vi "Test1_5b.vi"(0 "Instrument VISA in":T1={"AWG VISA"="81160A", "Oscilloscope  VISA "="DSO80204B", "Integration Board IP"="172.16.7.43", "connection ID"=refnum, "report out"=refnum}, 2 "Report Enable":bool, 5 "L1 version":bool, 9 "Cycles Burst":i32=10000, 11 "error in":errorcluster) -> (4 "Instrument VISA out":T1={"AWG VISA"="81160A", "Oscilloscope  VISA "="DSO80204B", "Integration Board IP"="172.16.7.43", "connection ID"=refnum, "report out"=refnum}, 6 "DT_50_L0":i32[][](array[numeric]), 8 "L1 Level Above Noise":i32, 15 "error out":errorcluster)   [LabVIEW 2009]
doc: "This VI helps in the comparison between the sum of different channels."
uses:
  <instrlib>/Agilent 81150/Agilent 81150.lvlib
  <vilib>/Analysis/NI_AALPro.lvlib
  <vilib>/Utility/NIReport.llb/NI_report.lvclass
panel:
  out "XY Graph":cluster{"Y":dbl[], "Y":dbl[]}[](graph)
  out "IPR_Address":i32
  out "L1 Address":i32=17
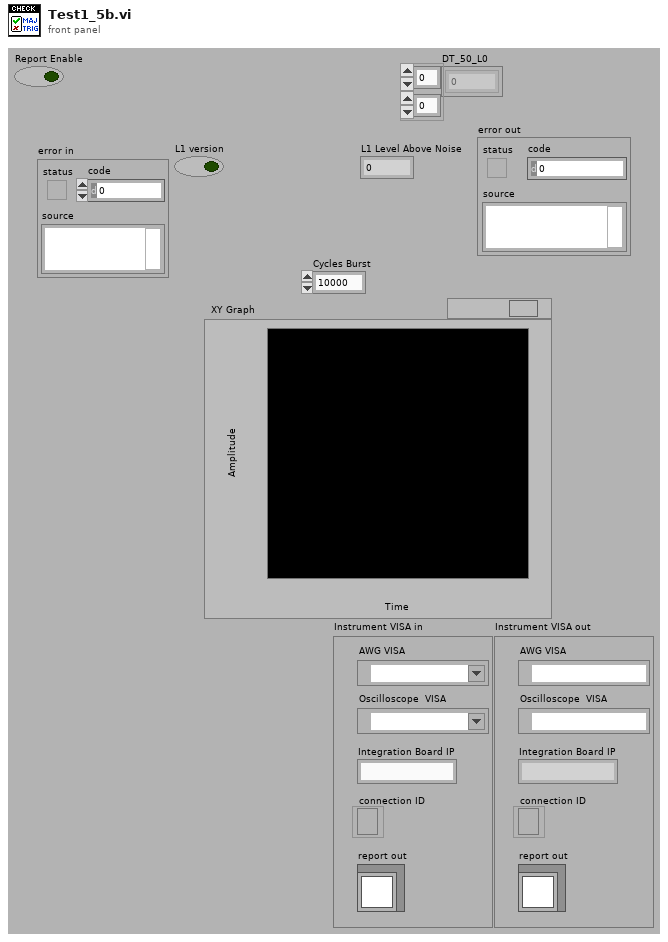
[diagram p1: front panel]
types:
  T1 = cluster{"AWG VISA":refnum<visa-resource-name>, "Oscilloscope  VISA ":refnum<visa-resource-name>, "Integration Board IP":string, "connection ID":refnum<k5>, "report out":refnum<class "NI_report.lvclass">}
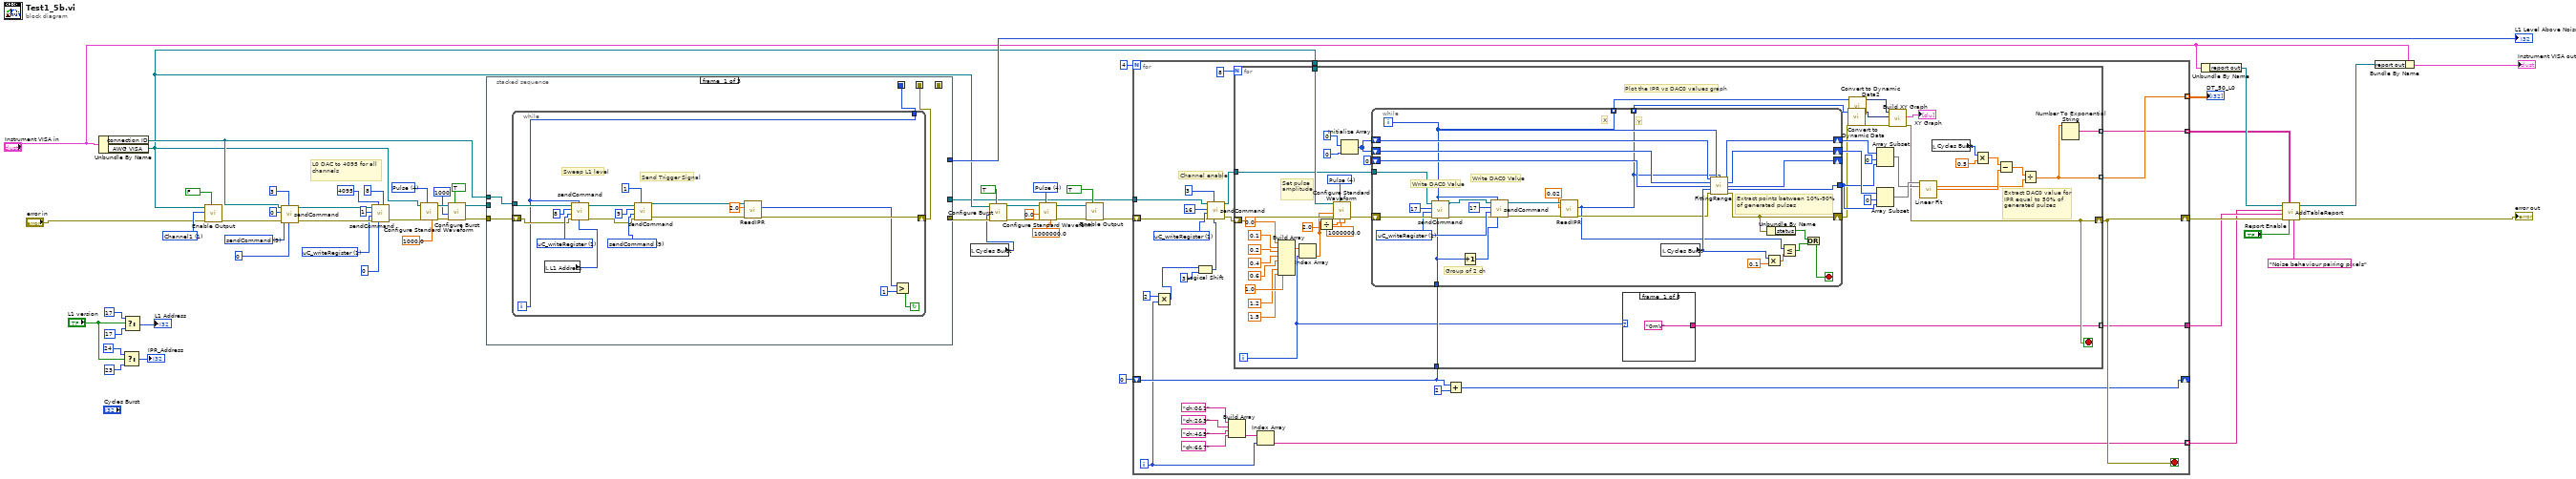
[diagram p0: block diagram]
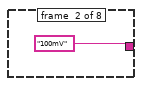
[diagram p2: hidden frame]
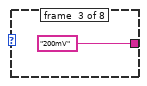
[diagram p3: hidden frame]
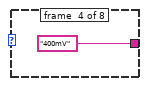
[diagram p4: hidden frame]
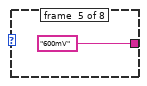
[diagram p5: hidden frame]
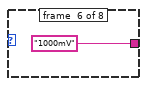
[diagram p6: hidden frame]
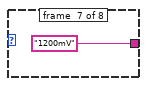
[diagram p7: hidden frame]
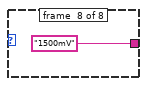
[diagram p8: hidden frame]
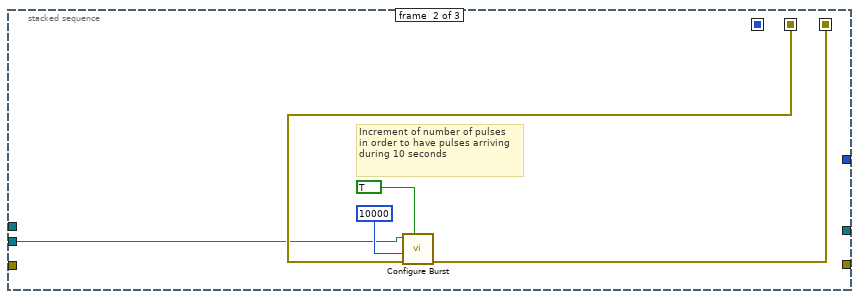
[diagram p9: hidden frame]
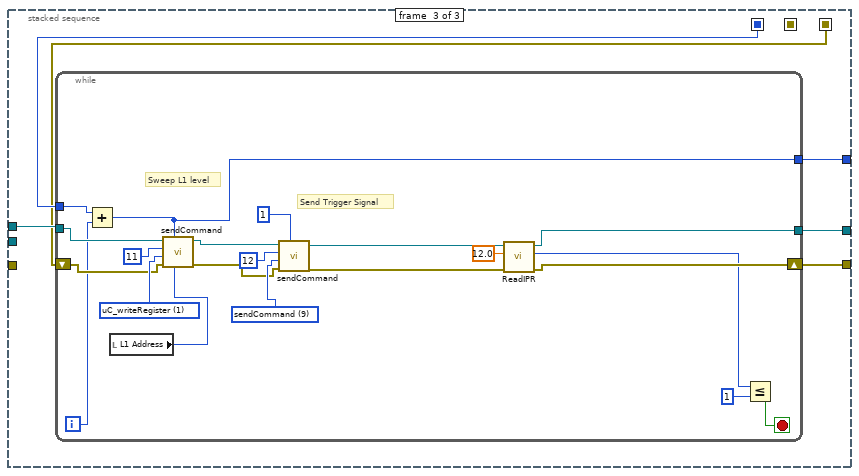
[diagram p10: hidden frame]
diagram:
  w28 = u16 4 items=["Sine", "Square", "Ramp Up", "Ramp Down", "Pulse", "Noise", "DC"] ("Waveform (0: Sine)")
  w44 = u16 4 items=["Sine", "Square", "Ramp Up", "Ramp Down", "Pulse", "Noise", "DC"] ("Waveform (0: Sine)")
  w51 = u16 1 items=["sendCommand"=9, "FPGA_writeRegister"=3, "FPGA_readRegister"=2, "uC_writeRegister"=1, "uC_readRegister"=0] ("Action")
  w58 = u16 9 items=["sendCommand"=9, "FPGA_writeRegister"=3, "FPGA_readRegister"=2, "uC_writeRegister"=1, "uC_readRegister"=0] ("Action")
  w60 = u16 1 items=["Channel1"=1, "Channel2"=2] ("Channel (1: Channel1)")
  # "L0 DAC to 4095 for all channels"
  n1 = Unbundle By Name("Instrument VISA in") -> ("connection ID"=w39:refnum<k5>, "AWG VISA"=w29:refnum<visa-resource-name>)
  n2 = Select(t=24 ("Address"), s="L1 version", f=23 ("Address")) -> (s? t:f=→"IPR_Address":i32)
  n3 = Select(t=17 ("Address"), s="L1 version", f=17 ("Address")) -> (s? t:f=→"L1 Address":i32)
  n4 = call <instrlib>:"Enable Output.vi"("Enable Output (T: Enable)"=FALSE, "error in (no error)"="error in", "Channel (1: Channel1)"=w60, "VISA resource name"=w29) -> ("error out"=w57:errorcluster)  [unwired: 6 in, 1 out]
  n5 = call "sendCommand.vi"("Address"=0, "Data"=3, "error in"=w57, "Action"=w58, "id_in"=0 ("id"), "connection ID"=w39) -> ("error out"=w53:errorcluster, "connection ID out"=w52:refnum<k5>)  [unwired: 1 in, 3 out]
  n6 = call "sendCommand.vi"("number data"=8, "Address"=0, "Data"=4095, "error in"=w53, "Action"=w51, "id_in"=1 ("id"), "connection ID"=w52) -> ("error out"=w46:errorcluster)  [unwired: 4 out]
  n7 = call <instrlib>:"Configure Standard Waveform.vi"("Frequency (1000.0 Hz)"=1000.0, "Waveform (0: Sine)"=w44, "error in (no error)"=w46, "VISA resource name"=w29) -> ("error out"=w43:errorcluster, "VISA resource name out"=w42:refnum<visa-resource-name>)  [unwired: 6 in]
  n8 = call <instrlib>:"Configure Burst.vi"("Enable Burst (F: Disable)"=TRUE, "error in (no error)"=w43, "Burst Count (2)"=1000, "VISA resource name"=w42) -> ("error out"=w40:errorcluster, "VISA resource name out"=w38:refnum<visa-resource-name>)  [unwired: 6 in]
  n9 = stacked-sequence {
    seq-local: [w63 _ _] -> [_ w87 _]
    seq-local: [w62 _ _] -> [_ _ w93]
    seq-local: [_ w86 _] -> [_ _ w92]
    tunnel: w40 -> [w65 _ _]
    tunnel: w39 -> [w64 _ w94]
    tunnel: w38 -> [_ w85 _]
    tunnel: [_ _ w91] -> w36
    tunnel: [_ _ w90] -> w30
    tunnel: [_ _ w89] -> w1
    frame #0 {
      n10 = while {
        tunnel: w64 -> [w75]
        tunnel: [w72] -> w62
        shift-right: [w68] -> w63
        shift-left: w65 -> [w76]
        i -> [w72]
        stop <- w79 continue-if-true
        w78 = u16 1 items=["sendCommand"=9, "FPGA_writeRegister"=3, "FPGA_readRegister"=2, "uC_writeRegister"=1, "uC_readRegister"=0] ("Action")
        w83 = u16 9 items=["sendCommand"=9, "FPGA_writeRegister"=3, "FPGA_readRegister"=2, "uC_writeRegister"=1, "uC_readRegister"=0] ("Action")
        # "Sweep L1 level"
        # "Send Trigger Signal"
        n11 = local read "L1 Address"() -> (w71:i32)
        n12 = call "sendCommand.vi"("Address"=w71, "Data"=w72, "error in"=w76, "Action"=w78, "id_in"=8 ("id"), "connection ID"=w75) -> ("error out"=w73:errorcluster, "connection ID out"=w74:refnum<k5>)  [unwired: 1 in, 3 out]
        n13 = call "sendCommand.vi"("Data"=1, "error in"=w73, "Action"=w83, "id_in"=9 ("id"), "connection ID"=w74) -> ("error out"=w70:errorcluster, "connection ID out"=w69:refnum<k5>)  [unwired: 2 in, 3 out]
        n14 = call "ReadIPR.vi"("error in"=w70, 10:2.0 ("Delay Time (s)"), "connection ID"=w69) -> ("error out"=w68:errorcluster, "IPR value"=w66:i32)  [unwired: 6 in, 1 out]
        n15 = Greater?(x=w66, y=1) -> (0:w79:bool)
      }
    }
    frame #1 {
      # "Increment of number of pulses    in order to have pulses arriving during 10 seconds"
      n16 = call <instrlib>:"Configure Burst.vi"("Enable Burst (F: Disable)"=TRUE, "error in (no error)"=w87, "Burst Count (2)"=10000, "VISA resource name"=w85) -> ("error out"=w86:errorcluster)  [unwired: 6 in, 1 out]
    }
    frame #2 {
      n17 = while {
        tunnel: w94 -> [w110]
        shift-right: [w98] -> w90
        shift-left: w92 -> [w111]
        tunnel: w93 -> [w109]
        tunnel: [w107] -> w91
        tunnel: [w95] -> w89
        i -> [w108]
        stop <- w114 stop-if-true
        w105 = u16 9 items=["sendCommand"=9, "FPGA_writeRegister"=3, "FPGA_readRegister"=2, "uC_writeRegister"=1, "uC_readRegister"=0] ("Action")
        w113 = u16 1 items=["sendCommand"=9, "FPGA_writeRegister"=3, "FPGA_readRegister"=2, "uC_writeRegister"=1, "uC_readRegister"=0] ("Action")
        # "Send Trigger Signal"
        # "Sweep L1 level"
        n18 = Add(x=w109, y=w108) -> (x+y=w107:i32)
        n19 = local read "L1 Address"() -> (w106:i32)
        n20 = call "sendCommand.vi"("Address"=w106, "Data"=w107, "error in"=w111, "Action"=w113, "id_in"=11 ("id"), "connection ID"=w110) -> ("error out"=w102:errorcluster, "connection ID out"=w101:refnum<k5>)  [unwired: 1 in, 3 out]
        n21 = call "sendCommand.vi"("Data"=1, "error in"=w102, "Action"=w105, "id_in"=12 ("id"), "connection ID"=w101) -> ("error out"=w100:errorcluster, "connection ID out"=w99:refnum<k5>)  [unwired: 2 in, 3 out]
        n22 = call "ReadIPR.vi"("error in"=w100, 10:12.0 ("Delay Time (s)"), "connection ID"=w99) -> ("error out"=w98:errorcluster, "IPR value"=w96:i32, "connection ID out"=w95:refnum<k5>)  [unwired: 6 in]
        n23 = Less Or Equal?(x=w96, y=1) -> (x <= y?=w114:bool)
      }
    }
  }
  "L1 Level Above Noise" <- w36
  n24 = local read "Cycles Burst"() -> (w15:i32)
  n25 = call <instrlib>:"Configure Burst.vi"("Enable Burst (F: Disable)"=TRUE, "error in (no error)"=w30, "Burst Count (2)"=w15, "VISA resource name"=w29) -> ("error out"=w25:errorcluster, "VISA resource name out"=w26:refnum<visa-resource-name>)  [unwired: 6 in]
  n26 = call <instrlib>:"Configure Standard Waveform.vi"("Frequency (1000.0 Hz)"=1000000.0, "Waveform (0: Sine)"=w28, "error in (no error)"=w25, "Amplitude (1.0 Vpp)"=0.0, "VISA resource name"=w26) -> ("error out"=w24:errorcluster, "VISA resource name out"=w23:refnum<visa-resource-name>)  [unwired: 5 in]
  n27 = call <instrlib>:"Enable Output.vi"("Enable Output (T: Enable)"=TRUE, "error in (no error)"=w24, "VISA resource name"=w23) -> ("error out"=w20:errorcluster)  [unwired: 7 in, 1 out]
  n28 = for {
    N: 4 -> [_]
    tunnel: w29 -> [w138]
    tunnel: [w136] -> w14 mode=indexing
    shift-right: [w134] -> w12
    shift-left: w20 -> [w139]
    shift-right: [w126] -> _
    shift-left: 0 ("x") -> [w128]
    tunnel: [w119] -> w2 mode=indexing
    tunnel: [w118] -> w4 mode=indexing
    tunnel: [w117] -> w3
    tunnel: w1 -> [w116]
    i -> [w124]
    stop <- w134 stop-if-true
    w142 = u16 1 items=["sendCommand"=9, "FPGA_writeRegister"=3, "FPGA_readRegister"=2, "uC_writeRegister"=1, "uC_readRegister"=0] ("Action")
    # "Channel enable"
    n29 = Multiply(x=2, y=w124) -> (x*y=w132:i32)
    n30 = Logical Shift(y=w132, x=i16 3) -> (x << y=w129:i16)
    n31 = call "sendCommand.vi"("Address"=w129, "Data"=3, "error in"=w139, "Action"=w142, "id_in"=16 ("id"), "connection ID"=w116) -> ("error out"=w135:errorcluster, "connection ID out"=w133:refnum<k5>)  [unwired: 1 in, 3 out]
    n32 = Build Array("ch:0&1" ("search string/char (-)"), "ch:2&3" ("search string/char (-)"), "ch:4&5" ("search string/char (-)"), "ch:6&7" ("search string/char (-)")) -> (w125:string[])
    n33 = for {
      N: 8 -> [_]
      tunnel: w138 -> [w189]
      tunnel: w128 -> [w177]
      tunnel: [w149] -> w136 mode=indexing
      shift-right: [w151] -> w134
      shift-left: w135 -> [w152]
      tunnel: w133 -> [w150]
      tunnel: [w148] -> w118 mode=indexing
      tunnel: [w146] -> w117 mode=indexing
      i -> [w147]
      stop <- w151 stop-if-true
      w187 = u16 4 items=["Sine", "Square", "Ramp Up", "Ramp Down", "Pulse", "Noise", "DC"] ("Waveform (0: Sine)")
      # "Extract DAC0 value for IPR equal to 50% of generated pulses"
      # "Plot the IPR vs DAC0 values graph"
      # "Set pulse amplitude"
      n34 = Build Array(0.0 ("element"), 0.1 ("element"), 0.2 ("element"), 0.4 ("element"), 0.6 ("element"), 1.0 ("element"), 1.2 ("element"), 1.5 ("element")) -> (w178:dbl[])
      n35 = Index Array(array=w178, index=w147) -> (element=w144:dbl)
      n36 = Divide(x=w144, y=2.0) -> (x/y=w145:dbl)
      n37 = call <instrlib>:"Configure Standard Waveform.vi"("Frequency (1000.0 Hz)"=1000000.0, "DC Offset (0.0 Volts)"=w145, "Waveform (0: Sine)"=w187, "error in (no error)"=w152, "Amplitude (1.0 Vpp)"=w144, "VISA resource name"=w189) -> ("error out"=w176:errorcluster)  [unwired: 4 in, 1 out]
      n38 = Initialize Array(0 ("element"), 0 ("dimension size")) -> (w168:i32[])
      n39 = while {
        tunnel: w177 -> [w204]
        tunnel: [w198] -> w174 mode=indexing
        tunnel: [w205] -> w172 mode=indexing
        shift-right: [w222] -> w166
        shift-left: w168 -> [w220]
        shift-right: [w221] -> w165
        shift-left: w168 -> [w219]
        shift-right: [w212] -> w153
        shift-left: w176 -> [w225]
        shift-right: [w217] -> _
        shift-left: 0 ("Array Pointer out") -> [w218]
        tunnel: [w216] -> w162
        tunnel: w150 -> [w214]
        i -> [w205]
        stop <- w210 stop-if-true
        w208 = u16 1 items=["sendCommand"=9, "FPGA_writeRegister"=3, "FPGA_readRegister"=2, "uC_writeRegister"=1, "uC_readRegister"=0] ("Action")
        # "Group of 2 ch"
        # "Write DAC0 Value"
        # "Extract points between 10%-90% of generated pulses"
        # "Write DAC0 Value"
        # "Y"
        # "X"
        n40 = call "sendCommand.vi"("Address"=w204, "Data"=w205, "error in"=w225, "Action"=w208, "id_in"=17 ("id"), "connection ID"=w214) -> ("error out"=w207:errorcluster, "connection ID out"=w206:refnum<k5>)  [unwired: 1 in, 3 out]
        n41 = Increment(x=w204) -> (x+1=w203:i32)
        n42 = call "sendCommand.vi"("Address"=w203, "Data"=w205, "error in"=w207, "Action"=w208, "id_in"=17 ("id"), "connection ID"=w206) -> ("error out"=w202:errorcluster, "connection ID out"=w201:refnum<k5>)  [unwired: 1 in, 3 out]
        n43 = call "ReadIPR.vi"("error in"=w202, 10:0.02 ("Delay Time (s)"), "connection ID"=w201) -> ("error out"=w199:errorcluster, "IPR value"=w198:i32)  [unwired: 6 in, 1 out]
        n44 = local read "Cycles Burst"() -> (w215:i32)
        n45 = call "FittingRange.vi"("Array in (X)"=w220, "L0 DAC"=w205, "IPR"=w198, "Array in (Y)"=w219, "Array Pointer in"=w218, "Cycles Burst"=w215, "error in"=w199) -> ("Array out (X)"=w222:i32[], "Array out (Y)"=w221:i32[], "Array Pointer out"=w217:i32, "N_Array Elements"=w216:i32, "error out"=w212:errorcluster)  [unwired: 4 in]
        n46 = Multiply(x=w215, y=0.1) -> (x*y=w223:dbl)
        n47 = Unbundle By Name(w212) -> ("status"=w211:bool)
        n48 = Less Or Equal?(x=w198, y=w223) -> (x <= y?=w213:bool)
        n49 = Or(x=w211, y=w213) -> (x .or. y?=w210:bool)
      }
      n50 = case shown="0, Default" w147 {
        tunnel: ["0mV" ("regular expression") "100mV" ("regular expression") "200mV" ("regular expression") "400mV" ("regular expression") "600mV" ("regular expression") "1000mV" ("regular expression") "1200mV" ("regular expression") "1500mV" ("regular expression")] -> w146
        frame #0 {
        }
        frame #1 {
        }
        frame #2 {
        }
        frame #3 {
        }
        frame #4 {
        }
        frame #5 {
        }
        frame #6 {
        }
        frame #7 {
        }
      }
      n51 = call "Convert to Dynamic Data"("Array"=w174) -> ("Dynamic Data Type"=w173:dynamicdata)  [unwired: 3 in]
      n52 = call "Convert to Dynamic Data2"("Array"=w172) -> ("Dynamic Data Type"=w171:dynamicdata)  [unwired: 3 in]
      n53 = Array Subset(array=w165, index=0, length=w162) -> (w161:i32[])
      n54 = Array Subset(array=w166, index=0, length=w162) -> (w160:i32[])
      n55 = call "Build XY Graph"("error in (no error)"=w153, "Y Input"=w173, "X Input"=w171) -> ("error out"=w151:errorcluster, "XY Graph"=→"XY Graph":cluster{"Y":dbl[], "Y":dbl[]}[])  [unwired: 7 in]
      n56 = call <vilib>:"Linear Fit.vi"("Y"=w161, "X"=w160) -> ("slope"=w154:dbl, "intercept"=w156:dbl)  [unwired: 9 in, 3 out]
      n57 = local read "Cycles Burst"() -> (w159:i32)
      n58 = Multiply(x=w159, y=0.5) -> (x*y=w157:dbl)
      n59 = Subtract(x=w157, y=w156) -> (x-y=w155:dbl)
      n60 = Divide(x=w155, y=w154) -> (x/y=w149:dbl)
      n61 = Number To Exponential String(number=w149) -> (E-format string=w148:string)  [unwired: 3 in]
    }
    n62 = Index Array(array=w125, index=w124) -> (element=w119:string)
    n63 = Add(x=w128, y=2) -> (x+y=w126:i32)
  }
  "DT_50_L0" <- w14
  n64 = Unbundle By Name("Instrument VISA in") -> ("report out"=w10:refnum<class "NI_report.lvclass">)
  n65 = call "AddTableReport.vi"("Table title"="Noise behaviour pairing pixels", "Report Enable"="Report Enable", "Data"=w4, "error in"=w12, "Columns"=w3, "Rows"=w2, "report in"=w10) -> ("error out"=→"error out":errorcluster, "report out"=w7:refnum<class "NI_report.lvclass">)  [unwired: 3 in]
  n66 = Bundle By Name(cluster="Instrument VISA in", "report out"=w7) -> (→"Instrument VISA out":T1)
